vi "StateMachine.vi"() -> ()   [LabVIEW 2017, in "GP22_TDC_Arduinoed.lvlib"]
uses:
  GP22_TDC_Arduinoed.lvlib
  typedefs/State.ctl
  typedefs/Data.ctl
  <vilib>/Utility/file.llb/Write To Spreadsheet File (DBL).vi
  <vilib>/Analysis/NI_AALBase.lvlib
  <vilib>/Analysis/NI_AALPro.lvlib
panel:
  in  "VISA resource name":refnum<visa-resource-name>="COM6"
  in  "Exit":bool
  in  "Tab Control":T1(tab)
  in  "Start calibration":bool
  in  "Save data":bool
  in  "Number of calibration readings":i32=100
  out "Standard deviation":dbl format="%^_2g"
  out "Mean":dbl format="%^_4g"
  out "Calibration readings":dbl[](array[numeric])
  in  "Wait time (ms)":u32=10
  out "Progress":u8(slide) scale=0.0..100.0
  out "Calibration histogram":T2(graph)
  out "Freq / Hz":dbl format="%^#_6g"
  out "output / s":dbl format="%^#_6g"
  in  "Single Measurement":bool caption="Measure"
  out "output/s":dbl[](array[numeric]) format="%^#_6g"
  in  "Time / ms (30000)":u32=30000
  out "Size":i32
  out "Mean Freq / Hz":dbl format="%^#_6g"
  out "Frac. S.D.":dbl format="%^#_6e"
  out "Mean Time / s":dbl format="%^.3e"
  in  "Time between calibrations (ms)":u32=1000
  in  "Multiple Measurements":bool caption="Measure"
  out "Freq. histogram":T2(graph)
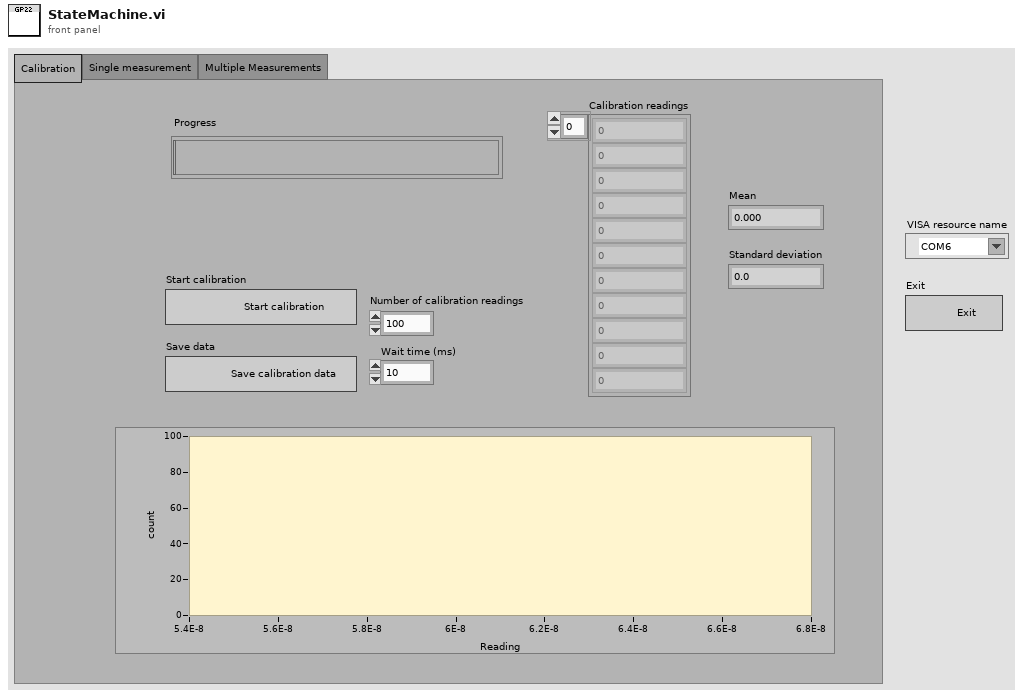
[diagram p1: front panel]
types:
  T1 = enum32{"Calibration", "Single measurement", "Multiple Measurements"}
  T2 = cluster{"X Values":dbl[], "Histogram: h(x)":i32[]}
  T3 = typedef "GP22_TDC_Arduinoed.lvlib/Data.ctl" = cluster{"VISA resource name":refnum<visa-resource-name>}
  T4 = typedef "GP22_TDC_Arduinoed.lvlib/State.ctl" = enum16{"Initialize", "Wait for Event", "Multiple Measurements", "Take calibration data", "Save calibration data", "Single measurement", "Exit"}
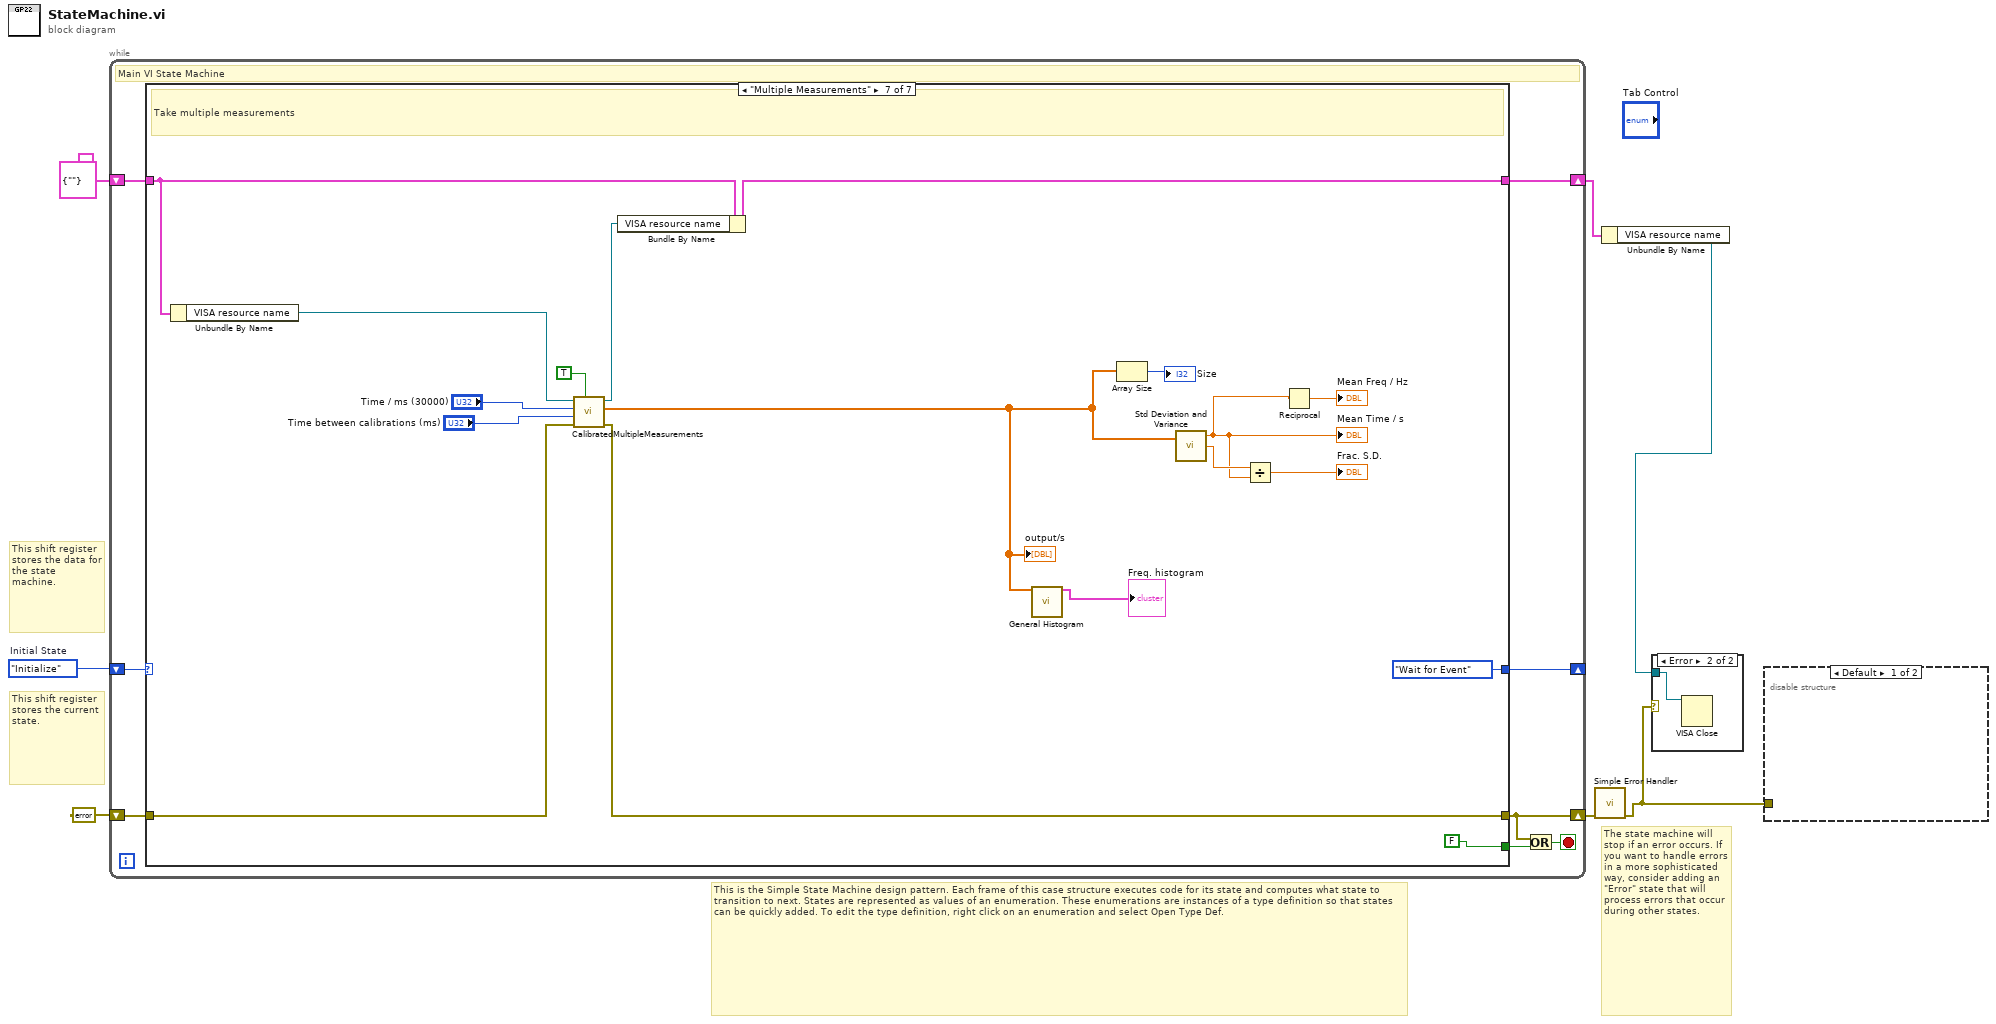
[diagram p0: block diagram]
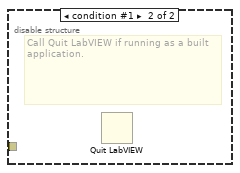
[diagram p3: hidden frame]
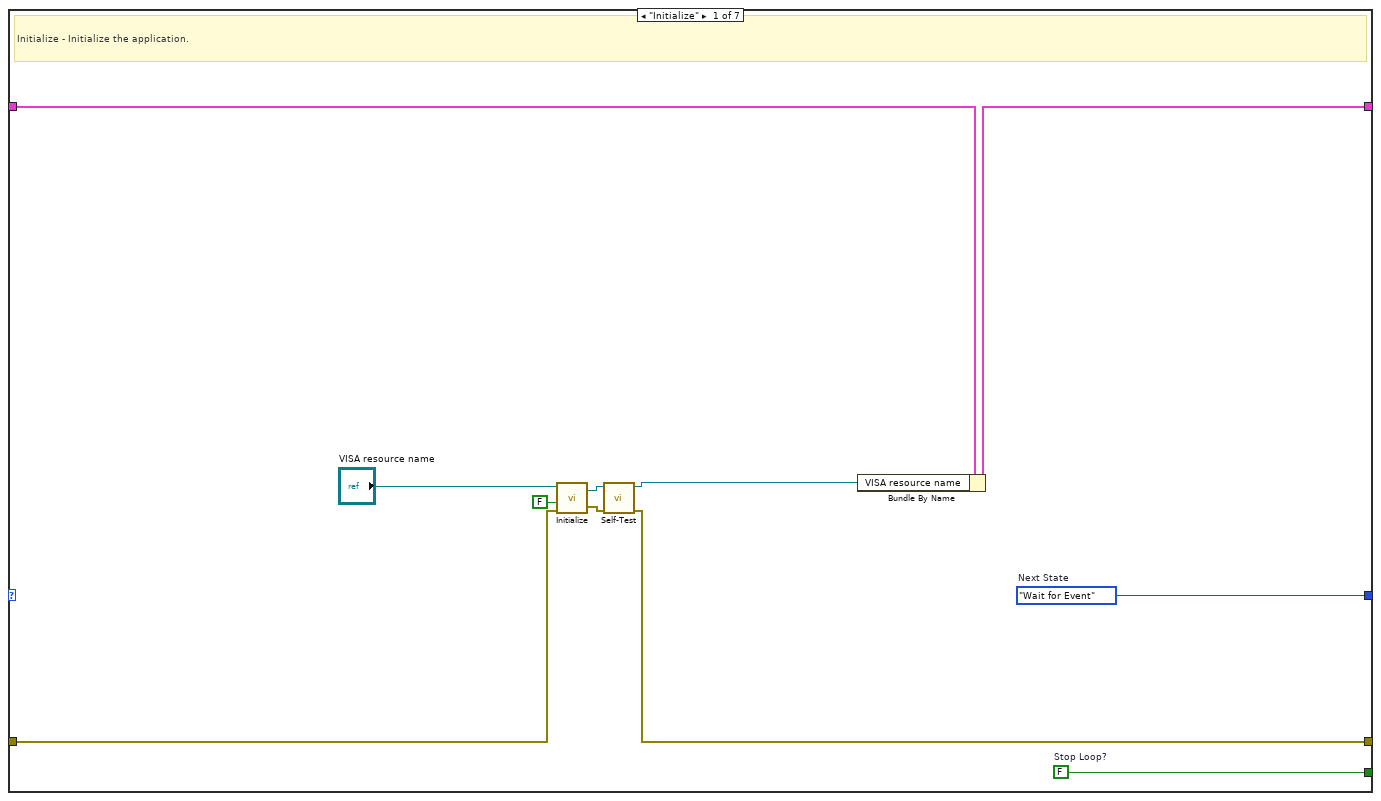
[diagram p4: hidden frame]
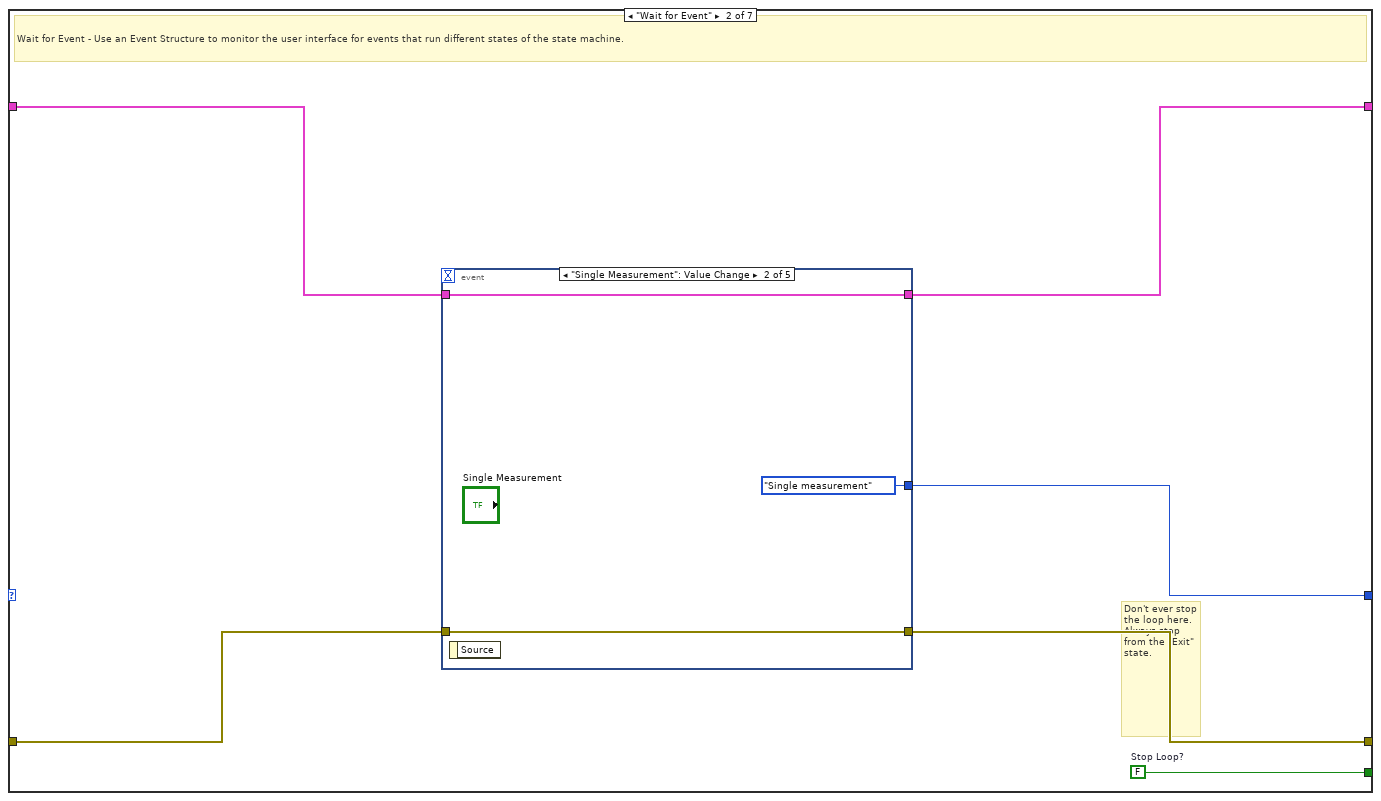
[diagram p5: hidden frame]
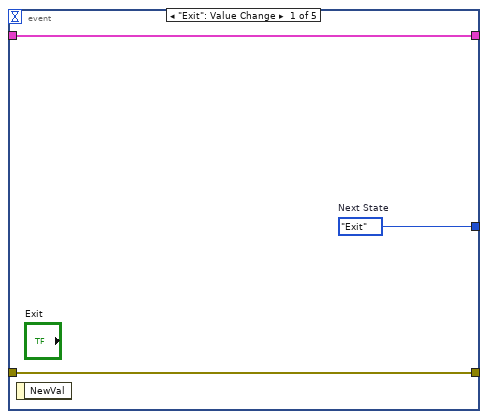
[diagram p6: hidden frame]
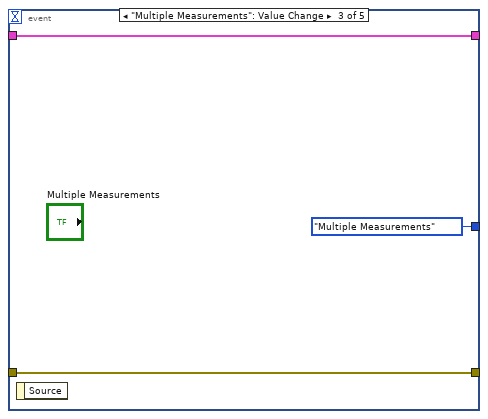
[diagram p7: hidden frame]
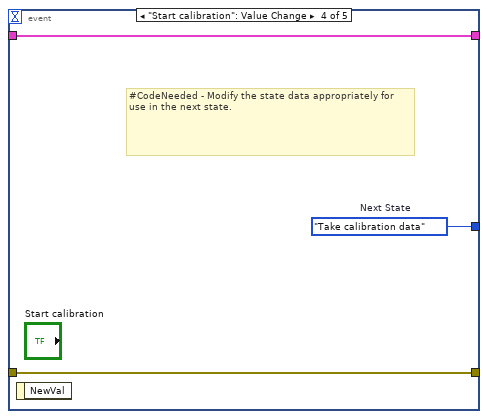
[diagram p8: hidden frame]
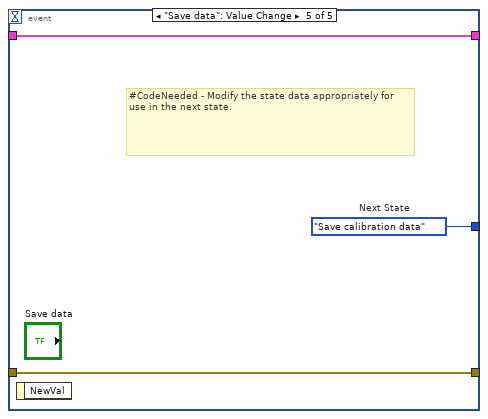
[diagram p9: hidden frame]
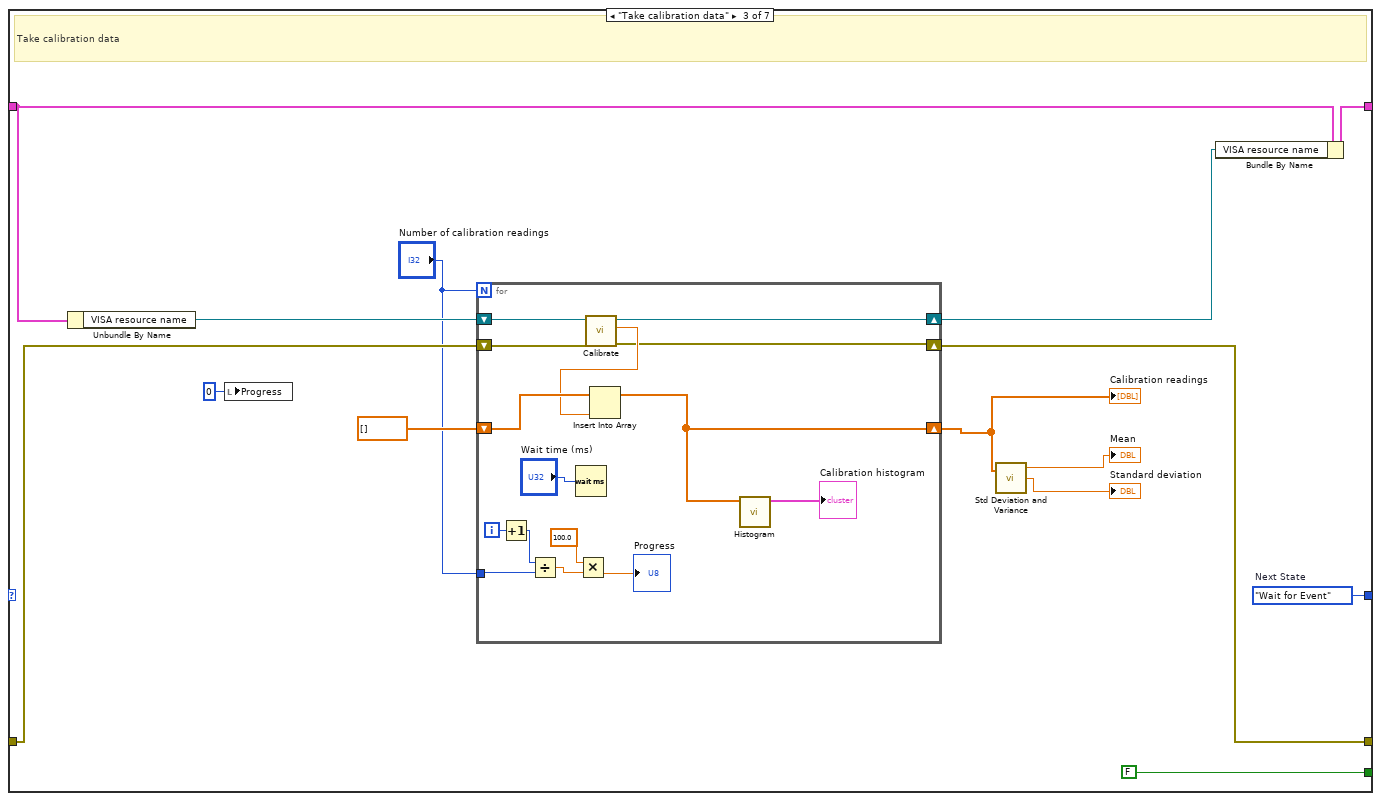
[diagram p10: hidden frame]
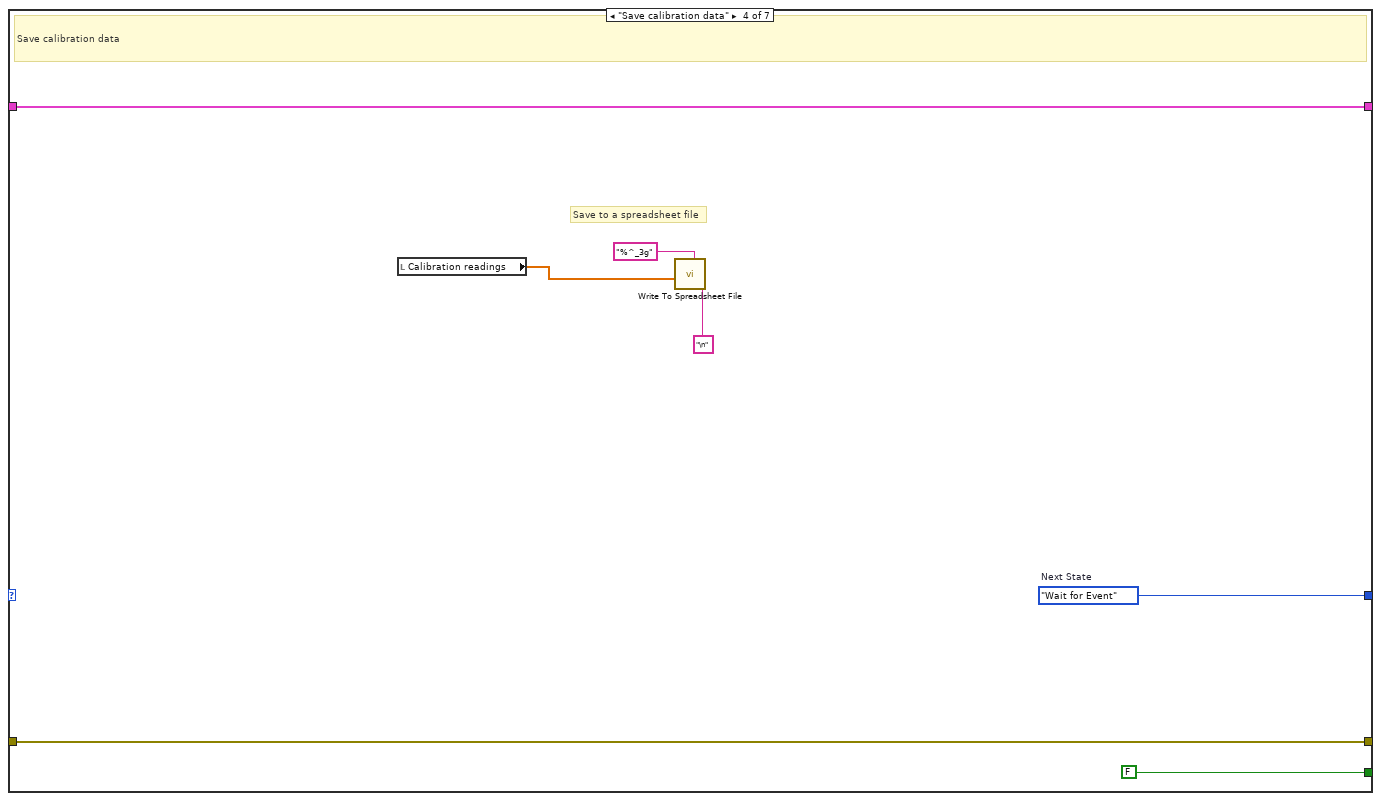
[diagram p11: hidden frame]
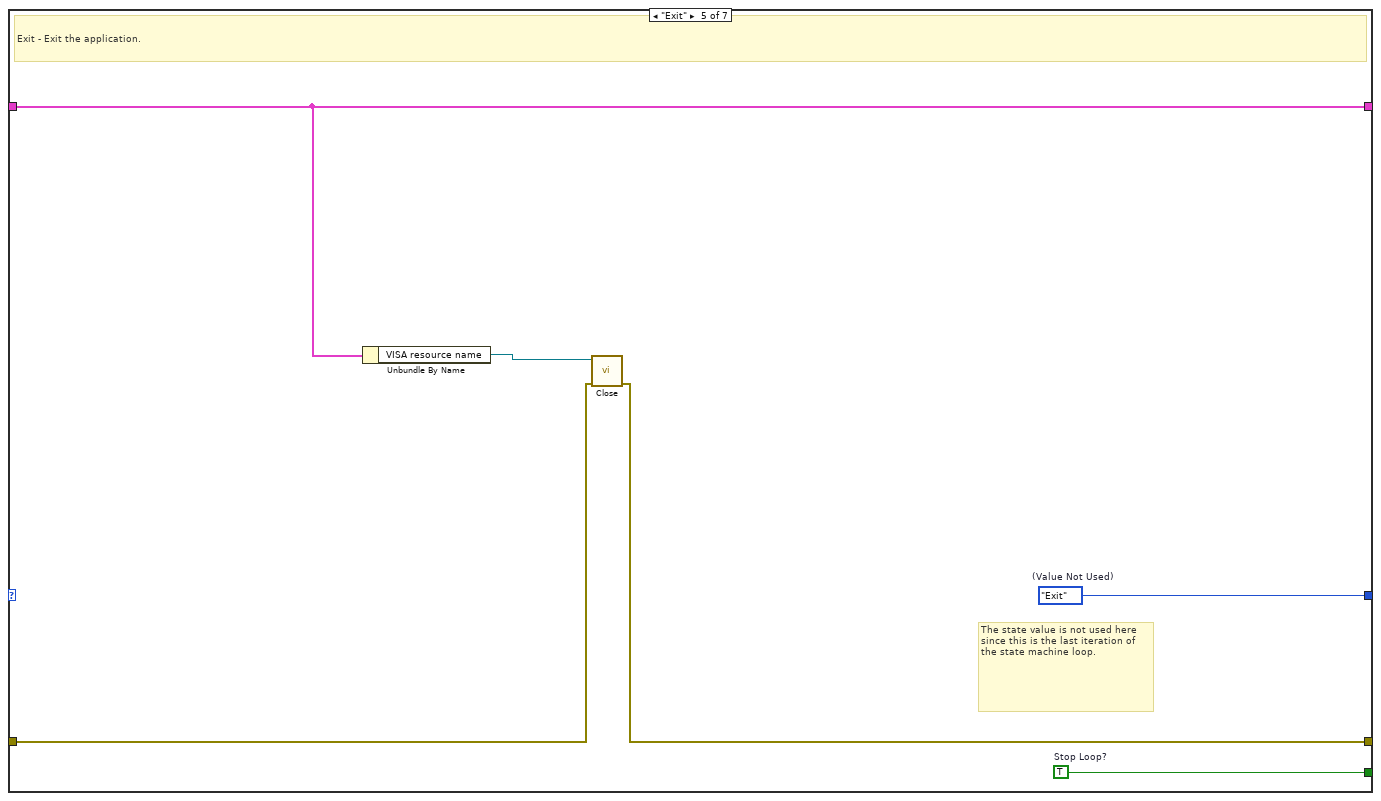
[diagram p12: hidden frame]
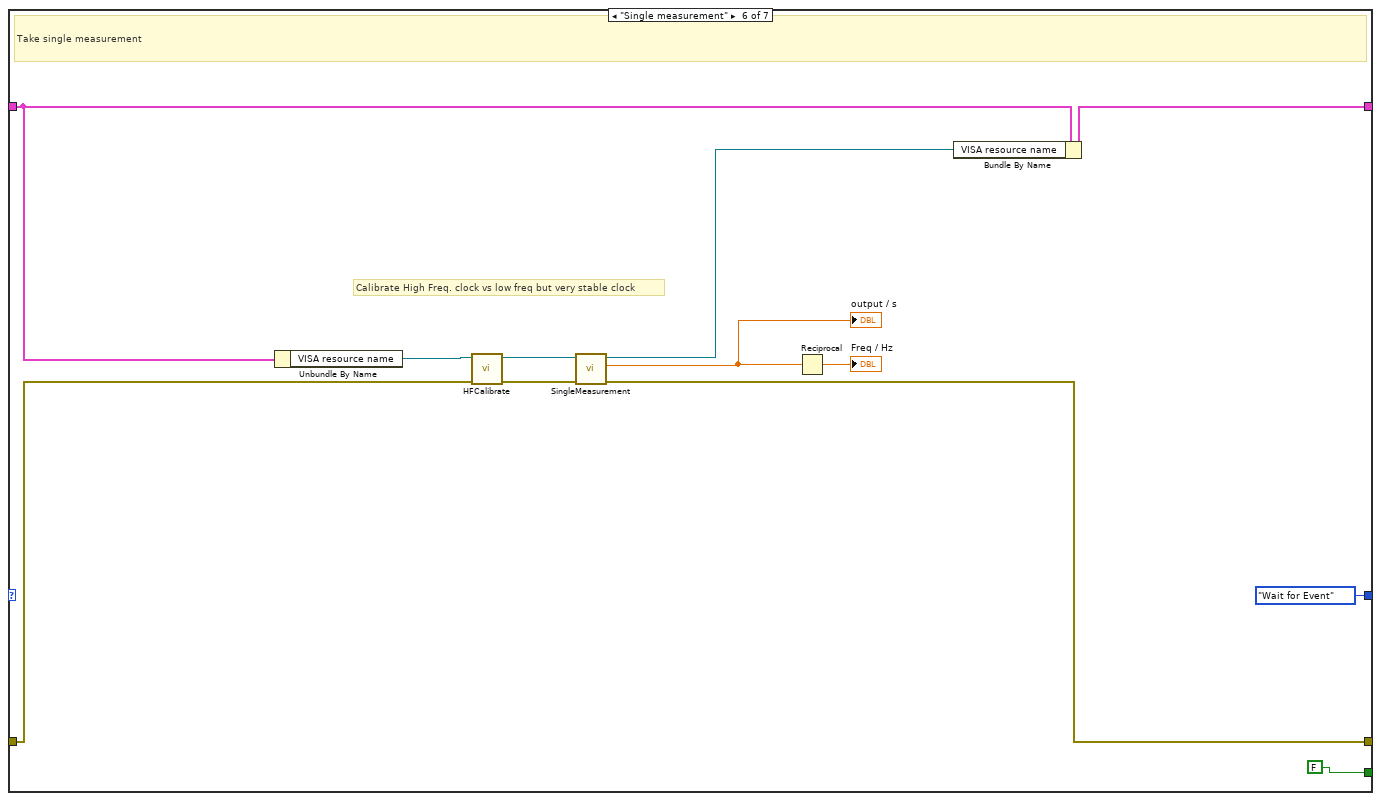
[diagram p13: hidden frame]
diagram:
  w7 = State."Initialize"  # Initial State
  # "The state machine will stop if an error occurs. If you want to handle errors in a more sophisticated way, consider adding an \"Error\" state that will process errors that occur during other states."
  # "This shift register stores the data for the state machine."
  # "This is the Simple State Machine design pattern. Each frame of this case structure executes code for its state and computes what state to transition to next. States are represented as values of an enumeration. These enumerations are instances of a type definition so that states can be quickly added. To edit the type definition, right click on an enumeration and select Open Type Def."
  # "This shift register stores the current state."
  n1 = while {
    shift-right: [w14] -> _
    shift-left: w7 -> [w15]
    shift-right: [w12] -> w3
    shift-left: T3 {"VISA resource name"=""} ("Data") -> [w13]
    shift-right: [w8] -> w4
    shift-left: errorcluster {"status"=FALSE, "code"=0, "source"=""} ("error constant") -> [w11]
    stop <- w9 stop-if-true
    # "Main VI State Machine"
    n2 = case shown="\"Multiple Measurements\"" w15 {
      tunnel: [w26 w32 w61 w83 w89 State."Wait for Event" ("(Value Not Used)") State."Wait for Event" ("(Value Not Used)")] -> w14
      tunnel: [w25 w31 FALSE ("Stop Loop?") FALSE ("Stop Loop?") w88 FALSE ("Stop Loop?") FALSE ("Stop Loop?")] -> w10
      tunnel: w13 -> [w24 w30 w58 w81 w87 w99 w119]
      tunnel: [w23 w29 w54 w81 w87 w98 w118] -> w12
      tunnel: w11 -> [w18 w28 w56 w80 w85 w90 w109]
      tunnel: [w17 w27 w55 w80 w84 w97 w105] -> w8
      frame "Initialize" {
        w25 = FALSE  # Stop Loop?
        w26 = State."Wait for Event"  # Next State
        # "Initialize - Initialize the application."
        n3 = call "Initialize.vi"("error in (no error)"=w18, "Default setup (True)"=FALSE, "VISA resource name"="VISA resource name") -> ("error out"=w19:errorcluster, "VISA resource name out"=w21:refnum<visa-resource-name>)  [unwired: 3 in]
        n4 = call "Self-Test.vi"("error in (no error)"=w19, "VISA resource name"=w21) -> ("error out"=w17:errorcluster, "VISA resource name out"=w20:refnum<visa-resource-name>)  [unwired: 6 in, 2 out]
        n5 = Bundle By Name(cluster=w24, "VISA resource name"=w20) -> (w23:T3)
      }
      frame "Wait for Event" {
        w31 = FALSE  # Stop Loop?
        # "Don't ever stop the loop here. Always stop from the \"Exit\" state."
        # "Wait for Event - Use an Event Structure to monitor the user interface for events that run different states of the state machine."
        n6 = event shown="[1] \"Single Measurement\": Value Change" {
          selector: _ -> [_ _ _ _ _]
          dyn-events: _ -> [_ _ _ _ _]
          timeout: _ -> [_ _ _ _ _]
          tunnel: [w35 State."Single measurement" ("Next State") State."Multiple Measurements" ("Next State") w44 w47] -> w32
          tunnel: w30 -> [w34 w38 w41 w42 w45]
          tunnel: [w34 w38 w41 w42 w45] -> w29
          tunnel: w28 -> [w33 w37 w40 w43 w46]
          tunnel: [w33 w37 w40 w43 w46] -> w27
          event "Exit": Value Change {
            w35 = State."Exit"  # Next State
            n7 = event-data() -> ()  [unwired: 1 in, 1 out]
          }
          event "Single Measurement": Value Change {
            n8 = event-data() -> ()  [unwired: 1 in, 1 out]
          }
          event "Multiple Measurements": Value Change {
            n9 = event-data() -> ()  [unwired: 1 in, 1 out]
          }
          event "Start calibration": Value Change {
            w44 = State."Take calibration data"  # Next State
            # "#CodeNeeded - Modify the state data appropriately for use in the next state."
            n10 = event-data() -> ()  [unwired: 1 in, 1 out]
          }
          event "Save data": Value Change {
            w47 = State."Save calibration data"  # Next State
            # "#CodeNeeded - Modify the state data appropriately for use in the next state."
            n11 = event-data() -> ()  [unwired: 1 in, 1 out]
          }
        }
      }
      frame "Take calibration data" {
        w61 = State."Wait for Event"  # Next State
        # "Take calibration data"
        n12 = Unbundle By Name(w58) -> ("VISA resource name"=w57:refnum<visa-resource-name>)
        n13 = local write "Progress"(u8 0 ("Progress")) -> ()
        n14 = for {
          N: "Number of calibration readings" -> [_]
          shift-right: [w63] -> w49
          shift-left: dbl[] [] -> [w73]
          shift-right: [w70] -> w55
          shift-left: w56 -> [w75]
          shift-right: [w71] -> w53
          shift-left: w57 -> [w76]
          tunnel: "Number of calibration readings" -> [w67]
          i -> [w68]
          n15 = Increment(x=w68) -> (x+1=w64:i32)
          n16 = Divide(x=w64, y=w67) -> (x/y=w69:dbl)
          n17 = Wait (ms)(milliseconds to wait="Wait time (ms)") -> ()  [unwired: 1 out]
          n18 = Multiply(x=100.0, y=w69) -> (x*y=→"Progress":dbl)
          n19 = call "Calibrate.vi"("error in (no error)"=w75, "VISA resource name"=w76) -> ("error out"=w70:errorcluster, "output / s"=w72:dbl, "VISA resource name out"=w71:refnum<visa-resource-name>)  [unwired: 5 in, 1 out]
          n20 = Insert Into Array(array=w73, new element=w72) -> (w63:dbl[])  [unwired: 1 in]
          n21 = call <vilib>:"Histogram.vi"("X"=w63) -> ("Histogram Graph"=→"Calibration histogram":T2)  [unwired: 7 in, 3 out]
        }
        "Calibration readings" <- w49
        n22 = call <vilib>:"Std Deviation and Variance.vi"("X"=w49) -> ("mean"=→"Mean":dbl, "standard deviation"=→"Standard deviation":dbl)  [unwired: 1 in, 1 out]
        n23 = Bundle By Name(cluster=w58, "VISA resource name"=w53) -> (w54:T3)
      }
      frame "Save calibration data" {
        w83 = State."Wait for Event"  # Next State
        # "Save to a spreadsheet file"
        # "Save calibration data"
        n24 = local read "Calibration readings"() -> (w79:dbl[])
        n25 = call-poly <vilib>:"Write To Spreadsheet File.vi"("delimiter (\\t)"="\n" ("delimiter (\\t)"), "format (%.3f)"="%^_3g", "1D data"=w79) -> ()  [unwired: 5 in, 1 out]
      }
      frame "Exit" {
        w88 = TRUE  # Stop Loop?
        w89 = State."Exit"  # (Value Not Used)
        # "The state value is not used here since this is the last iteration of the state machine loop."
        # "Exit - Exit the application."
        n26 = Unbundle By Name(w87) -> ("VISA resource name"=w86:refnum<visa-resource-name>)
        n27 = call "Close.vi"("error in (no error)"=w85, "VISA resource name"=w86) -> ("error out"=w84:errorcluster)  [unwired: 9 in]
      }
      frame "Single measurement" {
        # "Calibrate High Freq. clock vs low freq but very stable clock"
        # "Take single measurement"
        n28 = Unbundle By Name(w99) -> ("VISA resource name"=w93:refnum<visa-resource-name>)
        n29 = call "HFCalibrate.vi"("error in (no error)"=w90, "VISA resource name"=w93) -> ("error out"=w91:errorcluster, "VISA resource name out"=w92:refnum<visa-resource-name>)  [unwired: 5 in, 2 out]
        n30 = call "SingleMeasurement.vi"("error in (no error)"=w91, "VISA resource name"=w92) -> ("error out"=w97:errorcluster, "output / s"=w100:dbl, "VISA resource name out"=w96:refnum<visa-resource-name>)  [unwired: 7 in]
        "output / s" <- w100
        n31 = Reciprocal(x=w100) -> (1/x=→"Freq / Hz":dbl)
        n32 = Bundle By Name(cluster=w99, "VISA resource name"=w96) -> (w98:T3)
      }
      frame "Multiple Measurements" {
        # "Take multiple measurements"
        n33 = Unbundle By Name(w119) -> ("VISA resource name"=w110:refnum<visa-resource-name>)
        n34 = call "CalibratedMultipleMeasurements.vi"("Show on call?"=TRUE, "error in"=w109, "Time between calibrations (ms)"="Time between calibrations (ms)", "Time / ms (30000)"="Time / ms (30000)", "VISA resource name"=w110) -> ("error out"=w105:errorcluster, "Times / s"=w103:dbl[], "VISA resource name out"=w106:refnum<visa-resource-name>)  [unwired: 3 in, 1 out]
        "output/s" <- w103
        n35 = Bundle By Name(cluster=w119, "VISA resource name"=w106) -> (w118:T3)
        n36 = call <vilib>:"General Histogram.vi"("X"=w103) -> ("Histogram Graph"=→"Freq. histogram":T2)  [unwired: 10 in, 4 out]
        n37 = Array Size(array=w103) -> (size(s)=→"Size":i32)
        n38 = call <vilib>:"Std Deviation and Variance.vi"("X"=w103) -> ("mean"=w111:dbl, "standard deviation"=w113:dbl)  [unwired: 1 in, 1 out]
        "Mean Time / s" <- w111
        n39 = Divide(x=w113, y=w111) -> (x/y=→"Frac. S.D.":dbl)
        n40 = Reciprocal(x=w111) -> (1/x=→"Mean Freq / Hz":dbl)
      }
    }
    n41 = Or(x=w8, y=w10) -> (x .or. y?=w9:bool)
  }
  n42 = call <vilib>:"Simple Error Handler.vi"("error in (no error)"=w4) -> ("error out"=w1:errorcluster)  [unwired: 4 in, 4 out]
  n43 = Unbundle By Name(w3) -> ("VISA resource name"=w2:refnum<visa-resource-name>)
  n44 = case shown="Error" w1 {
    tunnel: w2 -> [_ w120]
    frame No Error {
    }
    frame Error {
      n45 = VISA Close(VISA resource name=w120) -> ()  [unwired: 1 in, 1 out]
    }
  }
  n46 = disable-structure shown="Default" {
    disable-tunnel: w1 -> [_ _]
    frame condition #0 (active) {
    }
    frame condition #1 {
      # "Call Quit LabVIEW if running as a built application."
      n47 = Quit LabVIEW() -> ()  [unwired: 1 in]
    }
  }
